vi "Set Port Status.vi"(8 "error in (no error)":errorcluster, 9 "Valor HEX":string, 10 "Puerto":string, 11 "UI Actor in":refnum<class "UI Actor.lvclass">) -> (0 "error out":errorcluster, 3 "UI Actor out":refnum<class "UI Actor.lvclass">)   [LabVIEW 2020, in "UI Actor.lvlib" / "UI Actor.lvclass"]
uses:
  UI Actor.lvclass
  UI Actor.lvclass/UI Actor.ctl
  Abstract/Serial Device/Serial Device.lvclass
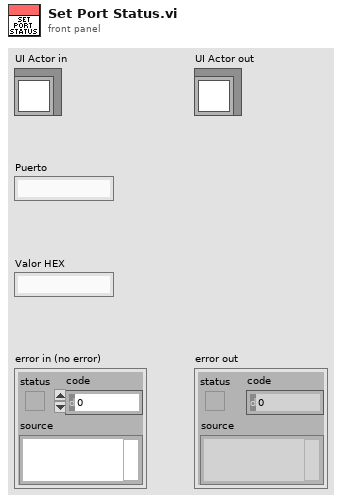
[diagram p1: front panel]
types:
  T1 = typedef "Control 1.ctl" = string
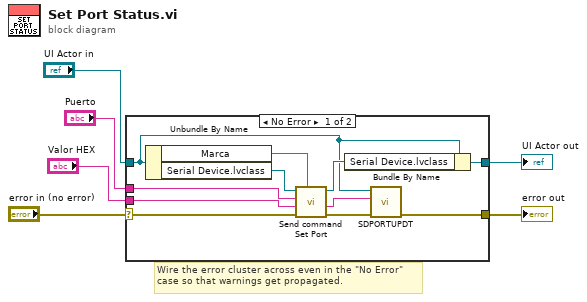
[diagram p0: block diagram]
diagram:
  # "Wire the error cluster across even in the \"No Error\"\ncase so that warnings get propagated."
  n1 = case shown="No Error" "error in (no error)" {
    selector: "error in (no error)" -> [w13 w19]
    tunnel: [w9 w19] -> w5
    tunnel: [w15 w18] -> w3
    tunnel: "UI Actor in" -> [w12 w18]
    tunnel: "Puerto" -> [w8 _]
    tunnel: "Valor HEX" -> [w7 _]
    frame No Error {
      n2 = Unbundle By Name(w12) -> ("Marca"=w16:T1, "Serial Device.lvclass"=w17:refnum<class "Serial Device.lvclass">)
      n3 = call-dynamic "Send command Set Port.vi"("Marca"=w16, "error in (no error)"=w13, "Valor HEX"=w7, "Puerto"=w8, "Serial Device in"=w17) -> ("error out"=w10:errorcluster, "Command"=w11:string, "Serial Device out"=w14:refnum<class "Serial Device.lvclass">)  [unwired: 3 in, 1 out]
      n4 = Bundle By Name(cluster=w12, "Serial Device.lvclass"=w14) -> (w15:refnum<class "UI Actor.lvclass">)
      n5 = call "SDPORTUPDT.vi"("error in (no error)"=w10, "Command"=w11, "UI Actor in"=w12) -> ("error out"=w9:errorcluster)  [unwired: 8 in]
    }
    frame Error {
    }
  }
  "error out" <- w5
  "UI Actor out" <- w3
